vi "Error Query.vi"(8 "error in (no error)":errorcluster, 11 "VISA resource name":refnum<visa-resource-name>) -> (0 "error out":errorcluster, 1 "Error Message":string, 2 "Error Code":i32[](array[numeric]), 3 "VISA resource name out":refnum<visa-resource-name>)   [LabVIEW 2024, in "EFmeter.lvlib"]
doc: "Queries the instrument for any errors in the instrument's error queue. It will continue to read errors until all errors have been read from the instrument. Any errors will be returned in the <B>error out</B> control.\n\n<B>Note:</B>\nThis VI is called automatically by most driver VIs so it is not usually necessary to call this in an application."
uses:
  EFmeter.lvlib
panel:
  # "EDIT: Note: The Error Query VI is included as a subVI in all driver VIs except low-level API VIs. If the instrument does not support error query, then remove the VI and remove subVI calls in each instrument driver VI that calls it."
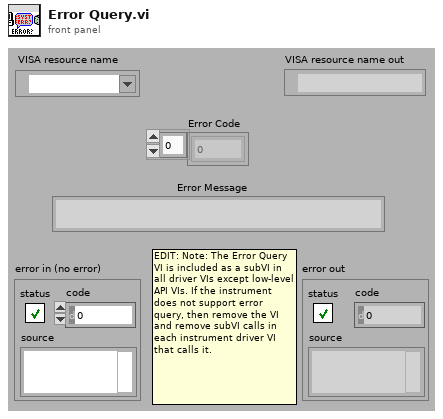
[diagram p1: front panel]
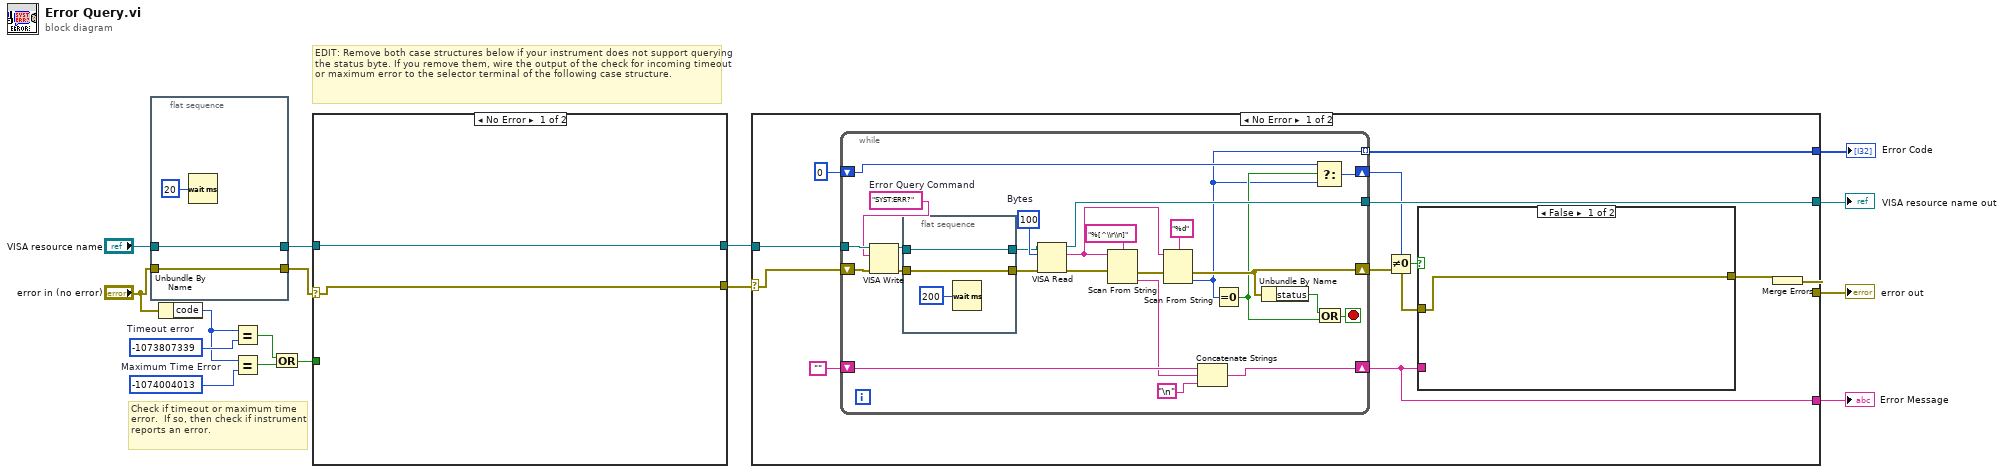
[diagram p0: block diagram]
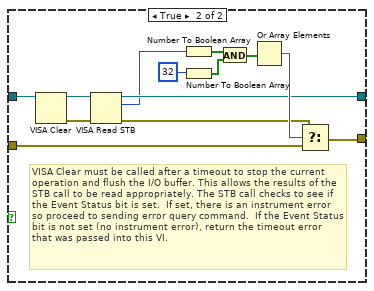
[diagram p3: hidden frame]
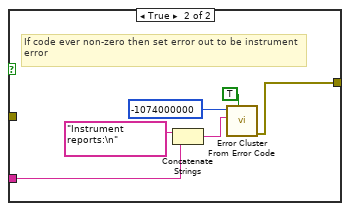
[diagram p4: hidden frame]
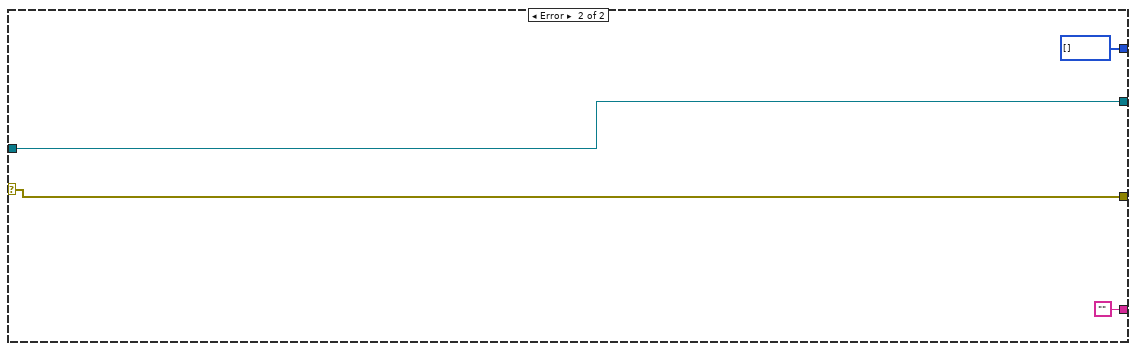
[diagram p5: hidden frame]
diagram:
  w8 = -1074004013  # Maximum Time Error
  w10 = -1073807339  # Timeout error
  # "Check if timeout or maximum time error.  If so, then check if instrument reports an error."
  # "EDIT: Remove both case structures below if your instrument does not support querying the status byte. If you remove them, wire the output of the check for incoming timeout or maximum error to the selector terminal of the following case structure."
  n1 = flat-sequence {
    tunnel: "VISA resource name" -> [w19]
    tunnel: [w19] -> w3
    tunnel: "error in (no error)" -> [w18]
    tunnel: [w18] -> w1
    frame #0 {
      n2 = Wait (ms)(milliseconds to wait=u32 20) -> ()  [unwired: 1 out]
    }
  }
  n3 = Unbundle By Name("error in (no error)") -> ("code"=w9:i32)
  n4 = Equal?(x=w9, y=w10) -> (x = y?=w6:bool)
  n5 = Equal?(x=w9, y=w8) -> (x = y?=w7:bool)
  n6 = Or(x=w6, y=w7) -> (x .or. y?=w5:bool)
  n7 = case shown="No Error" w1 {
    selector: w1 -> [w20 w24]
    tunnel: w3 -> [w21 w26]
    tunnel: [w21 w25] -> w11
    tunnel: [w20 w23] -> w12
    tunnel: w5 -> [_ w22]
    frame No Error {
    }
    frame Error {
      n8 = case shown="False" w22 {
        tunnel: w26 -> [w28 w34]
        tunnel: [w28 w31] -> w25
        tunnel: w24 -> [w27 w37]
        tunnel: [w27 w36] -> w23
        frame False {
          # "Error code not a timeout, so best to pass on to user."
        }
        frame True {
          # "VISA Clear must be called after a timeout to stop the current operation and flush the I/O buffer. This allows the results of the  STB call to be read appropriately. The STB call checks to see if the Event Status bit is set.  If set, there is an instrument error so proceed to sending error query command.  If the Event Status bit is not set (no instrument error), return the timeout error that was passed into this VI."
          n9 = VISA Clear(VISA resource name=w34) -> (VISA resource name out=w33:refnum<visa-resource-name>, error out=w32:errorcluster)  [unwired: 1 in]
          n10 = VISA Read STB(8:w32, 11:w33) -> (0:w30:errorcluster, 2:w29:u16, 3:w31:refnum<visa-resource-name>)
          n11 = Number To Boolean Array(number=w29) -> (Boolean array=w38:bool[])
          n12 = Number To Boolean Array(number=32) -> (Boolean array=w40:bool[])
          n13 = And(x=w38, y=w40) -> (x .and. y?=w39:bool[])
          n14 = Or Array Elements(Boolean array=w39) -> (logical OR=w35:bool)
          n15 = Select(t=w30, s=w35, f=w37) -> (s? t:f=w36:errorcluster)
        }
      }
    }
  }
  n16 = case shown="No Error" w12 {
    selector: w12 -> [w42 w89]
    tunnel: [w53 w92] -> w16
    tunnel: w11 -> [w52 w92]
    tunnel: [w50 w89] -> w15
    tunnel: [w45 ""] -> w14
    tunnel: [w44 i32[] []] -> w13
    frame No Error {
      n17 = while {
        tunnel: [w85] -> w53
        tunnel: w52 -> [w84]
        shift-right: [w74] -> w45
        shift-left: "" -> [w77]
        shift-right: [w72] -> w46
        shift-left: 0 -> [w73]
        shift-right: [w70] -> w43
        shift-left: w42 -> [w71]
        tunnel: [w65] -> w44 mode=indexing
        stop <- w80 stop-if-true
        w83 = u32 100  # Bytes
        w82 = "SYST:ERR?"  # Error Query Command
        n18 = VISA Write(VISA resource name=w84, write buffer=w82, error in (no error)=w71) -> (VISA resource name out=w61:refnum<visa-resource-name>, error out=w64:errorcluster)  [unwired: 1 out]
        n19 = flat-sequence {
          tunnel: w64 -> [w88]
          tunnel: [w88] -> w63
          tunnel: [w87] -> w62
          tunnel: w61 -> [w87]
          frame #0 {
            n20 = Wait (ms)(milliseconds to wait=u32 200) -> ()  [unwired: 1 out]
          }
        }
        n21 = VISA Read(VISA resource name=w62, byte count=w83, error in (no error)=w63) -> (VISA resource name out=w85:refnum<visa-resource-name>, read buffer=w78:string, error out=w69:errorcluster)  [unwired: 1 out]
        n22 = Scan From String(format string="%[^\\r\\n]", input string=w78, error in=w69) -> (error out=w68:errorcluster, output 1=w75:string)  [unwired: 2 in, 2 out]
        n23 = Scan From String(format string="%d", input string=w78, error in=w68) -> (error out=w70:errorcluster, output 1=w65:i32)  [unwired: 2 in, 2 out]
        n24 = Concatenate Strings(w77, w75, "\n") -> (w74:string)
        n25 = Equal To 0?(x=w65) -> (x = 0?=w66:bool)
        n26 = Unbundle By Name(w70) -> ("status"=w67:bool)
        n27 = Select(t=w73, s=w66, f=w65) -> (s? t:f=w72:i32)
        n28 = Or(x=w67, y=w66) -> (x .or. y?=w80:bool)
      }
      n29 = Not Equal To 0?(x=w46) -> (x != 0?=w48:bool)
      n30 = case shown="False" w48 {
        tunnel: w45 -> [_ w59]
        tunnel: [w54 w55] -> w47
        tunnel: w43 -> [w54 _]
        frame False {
        }
        frame True {
          # "If code ever non-zero then set error out to be instrument error"
          n31 = Concatenate Strings("Instrument reports:\n" ("Source"), w59) -> (w56:string)
          n32 = call <vilib>:"Error Cluster From Error Code.vi"("show call chain? (False)"=TRUE, "error message (\"\")"=w56, "error code (0)"=-1074000000 ("Code")) -> ("error out"=w55:errorcluster)  [unwired: 6 in]
        }
      }
      n33 = Merge Errors(w47) -> (w50:errorcluster)
    }
    frame Error {
    }
  }
  "VISA resource name out" <- w16
  "error out" <- w15
  "Error Message" <- w14
  "Error Code" <- w13
